vi "Open Examples.vi"   [LabVIEW 2023, in "MVC Actors.lvlib"]
doc: "Run this VI to open the MVC Actors Examples"
uses:
  MVC Actors.lvlib
panel:
  # "Run this VI to open the MVC Actors Examples"
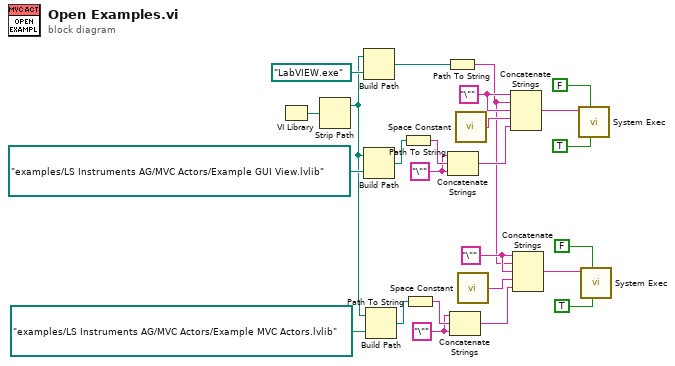
[diagram p0: block diagram]
diagram:
  w9 = "\""
  w11 = "\""
  w19 = "\""
  w21 = "\""
  n1 = VI Library() -> (path=w25:path)
  n2 = Strip Path(path=w25) -> (stripped path=w1:path)  [unwired: 1 out]
  n3 = Build Path(base path=w1, name or relative path=path "LabVIEW.exe") -> (appended path=w22:path)
  n4 = Build Path(base path=w1, name or relative path=path "examples/LS Instruments AG/MVC Actors/Example GUI View.lvlib") -> (appended path=w18:path)
  n5 = Build Path(base path=w1, name or relative path=path "examples/LS Instruments AG/MVC Actors/Example MVC Actors.lvlib") -> (appended path=w8:path)
  n6 = Path To String(path=w18) -> (string=w20:string)
  n7 = Path To String(path=w8) -> (string=w10:string)
  n8 = Path To String(path=w22) -> (string=w2:string)
  n9 = Concatenate Strings(w19, w20, w19) -> (w16:string)
  n10 = Concatenate Strings(w9, w10, w9) -> (w6:string)
  n11 = call <vilib>:"Space Constant.vi"() -> ("String"=w17:string)
  n12 = call <vilib>:"Space Constant.vi"() -> ("String"=w7:string)
  n13 = Concatenate Strings(w21, w2, w21, w17, w16) -> (w15:string)
  n14 = Concatenate Strings(w11, w2, w11, w7, w6) -> (w5:string)
  n15 = call <vilib>:"System Exec.vi"("run minimized? (F)"=TRUE, "wait until completion? (T)"=FALSE, "command line"=w15) -> ()  [unwired: 5 in, 4 out]
  n16 = call <vilib>:"System Exec.vi"("run minimized? (F)"=TRUE, "wait until completion? (T)"=FALSE, "command line"=w5) -> ()  [unwired: 5 in, 4 out]
